vi "Write Button.vi"(6 "Button":u16, 11 "Handle Drop Msg in":refnum<class "Handle Drop Msg.lvclass">) -> (3 "Handle Drop Msg out":refnum<class "Handle Drop Msg.lvclass">)   [LabVIEW 2017, in "Handle Drop Msg.lvclass"]
uses:
  <vilib>/gpm_packages/@cs/Test-executive-builder/Source/Test Executive Builder View/Test Executive Builder View Messages/Handle Drop Msg/Handle Drop Msg.lvclass
  <vilib>/gpm_packages/@cs/Test-executive-builder/Source/Test Executive Builder View/Test Executive Builder View Messages/Handle Drop Msg/Handle Drop Msg.lvclass/Handle Drop Msg.ctl
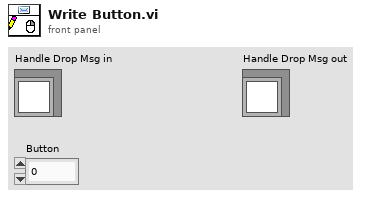
[diagram p1: front panel]
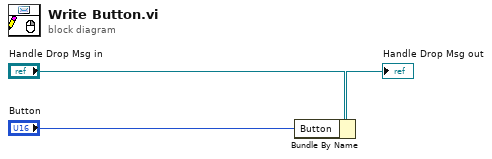
[diagram p0: block diagram]
diagram:
  n1 = Bundle By Name(cluster="Handle Drop Msg in", "Button"="Button") -> (→"Handle Drop Msg out":refnum<class "Handle Drop Msg.lvclass">)
